vi "Get Parent Path.vi"(11 "Node Path":string) -> (1 "Progressive Paths":string[](array[string]), 2 "Node Name":string, 3 "Parent Path":string)   [LabVIEW 2020, in "Tree Map.lvlib"]
doc: "Given a branch path strip it to return the parent path of specified branch and the name of the branch.\n\n<b>Author:</b> Piotr Kruczkowski <PrimaryKey>\n<b>License:</b> NewBSD\n\nCopyright (c) 2019, National Instruments\nAll rights reserved.\n\nRedistribution and use in source and binary forms, with or without\nmodification, are permitted provided that the following conditions are met:\n1. Redistributions of source code must retain the above copyright\n notice, this list of conditions and the following disclaimer.\n2. Redistributions in binary form must reproduce the above copyright\n notice, this list of conditions and the following disclaimer in the\n documentation and/or other materials provided with the distribution.\n3. Neither the name of National Instruments nor the\n names of its contributors may be used to endorse or promote products\n derived from this software without specific prior written permission.\n\nTHIS SOFTWARE IS PROVIDED BY National Instruments ''AS IS'' AND ANY\nEXPRESS OR IMPLIED WARRANTIES, INCLUDING, BUT NOT LIMITED TO, THE IMPLIED\nWARRANTIES OF MERCHANTABILITY AND FITNESS FOR A PARTICULAR PURPOSE ARE\nDISCLAIMED. IN NO EVENT SHALL National Instruments BE LIABLE FOR ANY\nDIRECT, INDIRECT, INCIDENTAL, SPECIAL, EXEMPLARY, OR CONSEQUENTIAL DAMAGES\n(INCLUDING, BUT NOT LIMITED TO, PROCUREMENT OF SUBSTITUTE GOODS OR SERVICES;\nLOSS OF USE, DATA, OR PROFITS; OR BUSINESS INTERRUPTION) HOWEVER CAUSED AND\nON ANY THEORY OF LIABILITY, WHETHER IN CONTRACT, STRICT LIABILITY, OR TORT\n(INCLUDING NEGLIGENCE OR OTHERWISE) ARISING IN ANY WAY OUT OF THE USE OF THIS\nSOFTWARE, EVEN IF ADVISED OF THE POSSIBILITY OF SUCH DAMAGE."
uses:
  Tree Map.lvlib
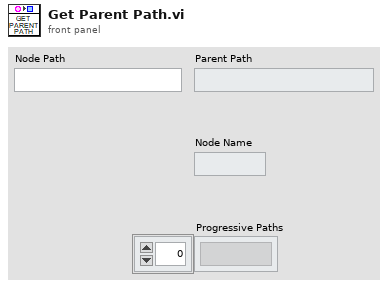
[diagram p1: front panel]
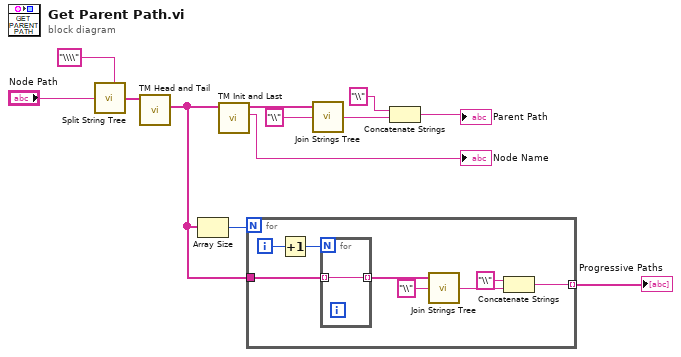
[diagram p0: block diagram]
diagram:
  n1 = call "Split String Tree.vi"("Split Pattern"="\\\\", "Input String"="Node Path") -> ("Split String"=w8:string[])  [unwired: 5 in]
  n2 = call "TM Head and Tail.vi"("List"=w8) -> ("Tail List"=w7:string[])  [unwired: 9 in, 1 out]
  n3 = Array Size(array=w7) -> (size(s)=w10:i32)
  n4 = call "TM Init and Last.vi"("List"=w7) -> ("Last"=→"Node Name":string, "Init List"=w6:string[])  [unwired: 9 in]
  n5 = for {
    N: w10 -> [_]
    tunnel: w7 -> [w18]
    tunnel: [w14] -> w9 mode=indexing
    i -> [w20]
    n6 = Increment(x=w20) -> (x+1=w19:i32)
    n7 = for {
      N: w19 -> [_]
      tunnel: w18 -> [w21] mode=indexing
      tunnel: [w21] -> w16 mode=indexing
    }
    n8 = call "Join Strings Tree.vi"("Separator"="\\" ("Separator (,)"), "Strings In"=w16) -> ("String"=w15:string)  [unwired: 1 in]
    n9 = Concatenate Strings("\\" ("string"), w15) -> (w14:string)
  }
  "Progressive Paths" <- w9
  n10 = call "Join Strings Tree.vi"("Separator"="\\" ("Separator (,)"), "Strings In"=w6) -> ("String"=w4:string)  [unwired: 1 in]
  n11 = Concatenate Strings("\\" ("Separator (,)"), w4) -> (→"Parent Path":string)
